vi "Point_Read_string.vi"(8 "Error In":errorcluster, 10 "Tag":string, 11 "Map":T1) -> (0 "Error Out":errorcluster, 1 "Value":string, 2 "Found?":bool, 3 "Map Out":T1, 4 "Time Stamp":timestamp, 5 "Valid?":bool)   [LabVIEW 2017, in "PointValueMap.lvlib"]
doc: "Gets the value of a map point."
uses:
  <vilib>/addons/PointValueMap/PointValueMap.lvlib
  <vilib>/addons/PointValueMap/controls/PointMap.ctl
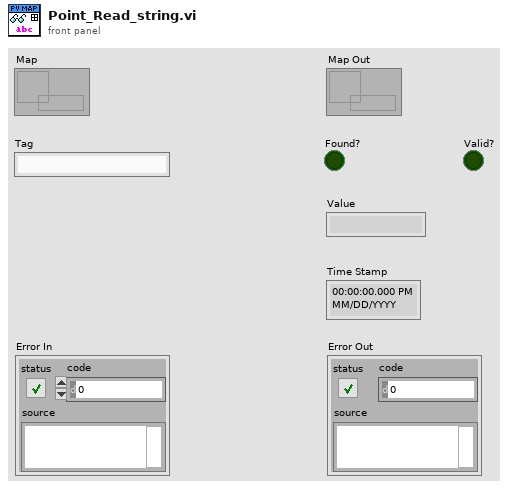
[diagram p1: front panel]
types:
  T1 = typedef "PointValueMap.lvlib/PointMap.ctl" = refnum<data-value>
  T2 = typedef "PointValueMap.lvlib/Point.ctl" = cluster{"Datatype":T3, "Timestamp":timestamp, "Value":variant, "Valid":bool}
  T3 = typedef "PointValueMap.lvlib/DataTypes.ctl" = enum16{"single", "double", "i32", "string", "variant"}
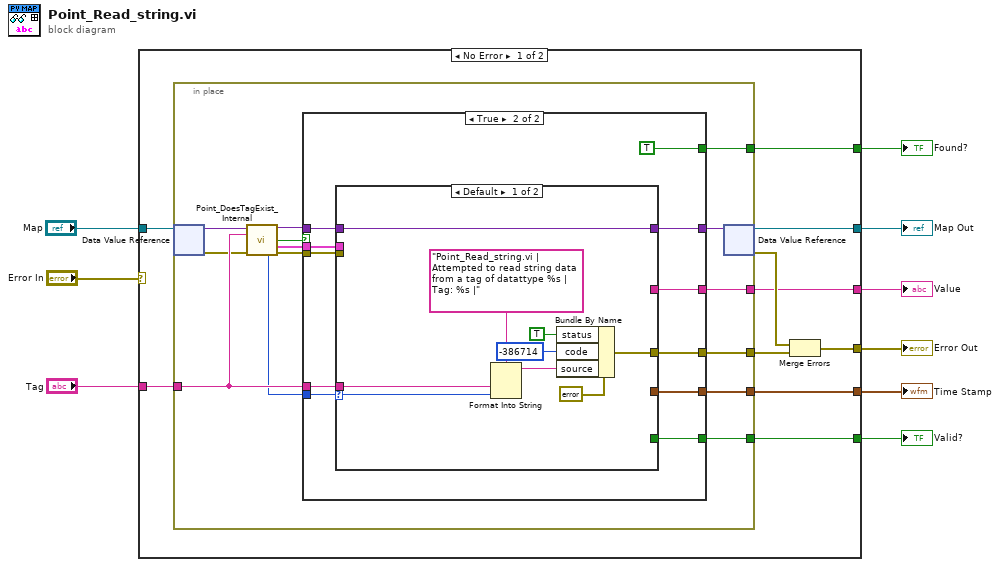
[diagram p0: block diagram]
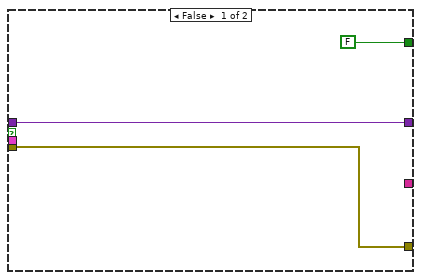
[diagram p2: hidden frame]
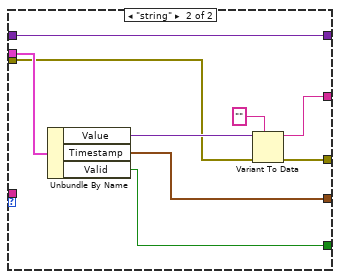
[diagram p3: hidden frame]
diagram:
  n1 = case shown="No Error" "Error In" {
    selector: "Error In" -> [_ w67]
    tunnel: "Map" -> [w19 w66]
    tunnel: "Tag" -> [w18 _]
    tunnel: [w15 w67] -> w8
    tunnel: [w14 _] -> w3
    tunnel: [w13 _] -> w6
    tunnel: [w12 w66] -> w4
    tunnel: [w11 _] -> w2
    tunnel: [w10 _] -> w1
    frame No Error {
      n2 = in-place {
        in-place-border: w18 -> [w28]
        in-place-border: [w32] -> w16
        in-place-border: [w31] -> w14
        in-place-border: [w30] -> w13
        in-place-border: [w21] -> w11
        in-place-border: [w20] -> w10
        n3 = in-place-dvr #1(w19) -> (w29:variant, w23:errorcluster)
        n4 = call <vilib>:"Point_DoesTagExist_Internal.vi"("Map"=w29, "Tag"=w28, "Error In"=w23) -> ("Map Out"=w25:variant, "Tag Exists"=w27:bool, "Point"=w22:T2, "Datatype"=w26:T3, "Error Out"=w24:errorcluster)  [unwired: 7 in, 1 out]
        n5 = case shown="True" w27 {
          tunnel: [w36 w47] -> w33
          tunnel: [w34 w46] -> w32
          tunnel: [_ w45] -> w31
          tunnel: [_ w44] -> w30
          tunnel: w25 -> [w36 w41]
          tunnel: w24 -> [w34 w40]
          tunnel: w28 -> [_ w43]
          tunnel: w26 -> [_ w42]
          tunnel: w22 -> [_ w39]
          tunnel: [_ w38] -> w21
          tunnel: [FALSE TRUE] -> w20
          frame False {
          }
          frame True {
            n6 = case shown="Default" w42 {
              selector: w42 -> [w48 _]
              tunnel: [w56 w65] -> w47
              tunnel: [w50 w59] -> w46
              tunnel: [_ w61] -> w45
              tunnel: w41 -> [w56 w65]
              tunnel: w40 -> [_ w60]
              tunnel: [_ w63] -> w44
              tunnel: w43 -> [w49 _]
              tunnel: w39 -> [_ w64]
              tunnel: [_ w57] -> w38
              frame Default {
                n7 = Format Into String(format string="Point_Read_string.vi | Attempted to read string data from a tag of datattype %s | Tag: %s |" ("source"), w49, w48) -> (resulting string=w52:string)  [unwired: 2 in, 1 out]
                n8 = Bundle By Name(cluster=errorcluster {"status"=FALSE, "code"=0, "source"=""} ("Error Out"), "status"=TRUE, "code"=-386714, "source"=w52) -> (w50:errorcluster)
              }
              frame "string" {
                n9 = Unbundle By Name(w64) -> ("Value"=w62:variant, "Timestamp"=w63:timestamp, "Valid"=w57:bool)
                n10 = Variant To Data(error in=w60, type="", Variant=w62) -> (data=w61:string, error out=w59:errorcluster)
              }
            }
          }
        }
        n11 = in-place-dvr #1(w33) -> (w12:T1, w17:errorcluster)
      }
      n12 = Merge Errors(w17, w16) -> (w15:errorcluster)
    }
    frame Error {
    }
  }
  "Error Out" <- w8
  "Time Stamp" <- w6
  "Map Out" <- w4
  "Value" <- w3
  "Valid?" <- w2
  "Found?" <- w1
